vi "svx_Colormap Frequency Lines.vi"(4 "pen":T2={"Width"=1, "Style"=enum."Solid"}, 5 "Frequency Type":dbl, 6 "color(black)":u32(colorbox), 7 "plot type":T4(ring), 8 "speed profile":cluster{"time [s]":dbl[], "speed [rpm]":dbl[]} {"speed [rpm]" format="%.2f"; "time [s]" format="%.2f"}, 9 "Range":T1, 10 "Plot Area:Size":T3, 11 "picture in":picture) -> (2 "Begin":cluster{"x":i16, "y":i16}, 3 "picture Out":picture)   [LabVIEW 2017, in "SVX Colormap.xctl"]
uses:
  <vilib>/addons/_XControls/Colormap/SVX Colormap.xctl
  <vilib>/Utility/miscctls.llb/LVBoundsTypeDef.ctl
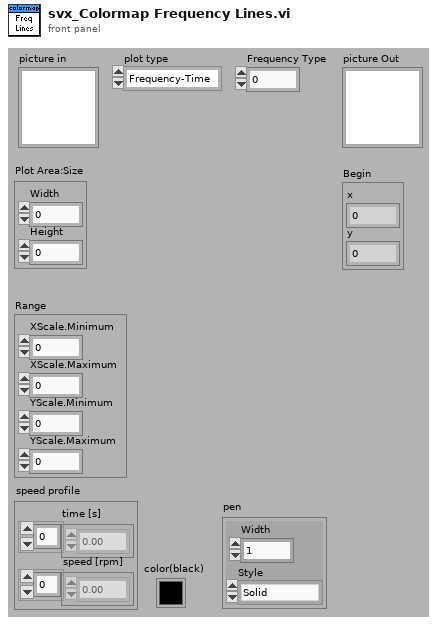
[diagram p1: front panel]
types:
  T1 = cluster{"XScale.Minimum":dbl, "XScale.Maximum":dbl, "YScale.Minimum":dbl, "YScale.Maximum":dbl}
  T2 = cluster{"Width":u16, "Style":enum32{"Solid", "Dash", "Dot", "DashDot", "DashDotDot"}}
  T3 = typedef "LVBoundsTypeDef.ctl" = cluster{"Width":u32, "Height":u32}
  T4 = enum16{"Frequency-Time", "Time-Frequency", "Order-Time", "Time-Order", "Frequency-RPM", "RPM-Frequency", "Order-RPM", "RPM-Order"}
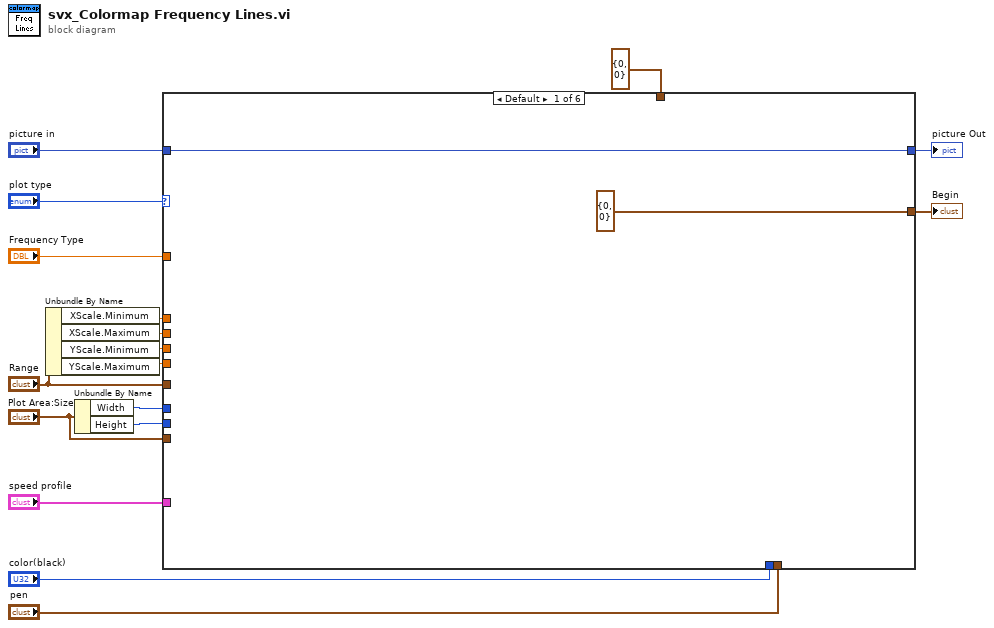
[diagram p0: block diagram]
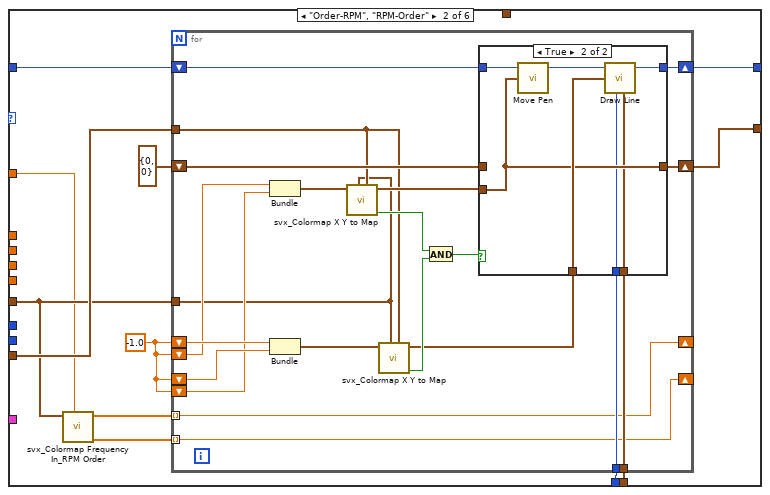
[diagram p2: hidden frame]
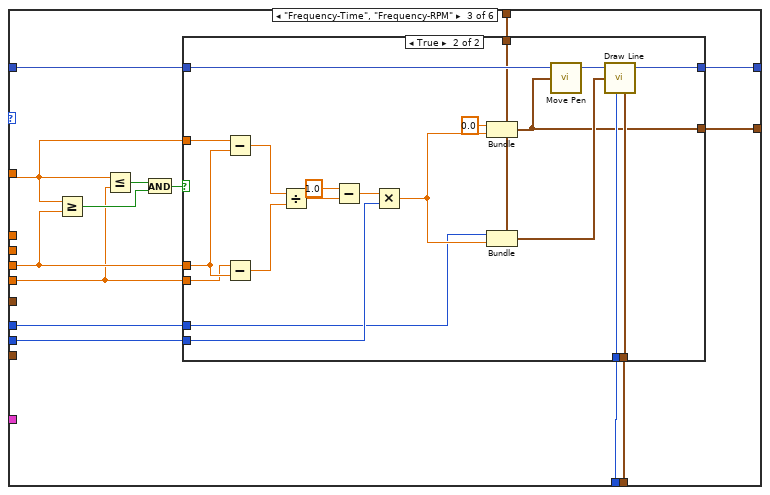
[diagram p4: hidden frame]
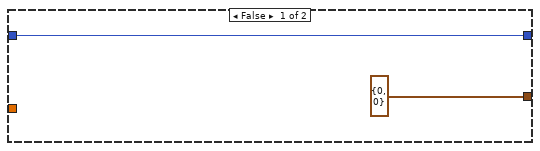
[diagram p5: hidden frame]
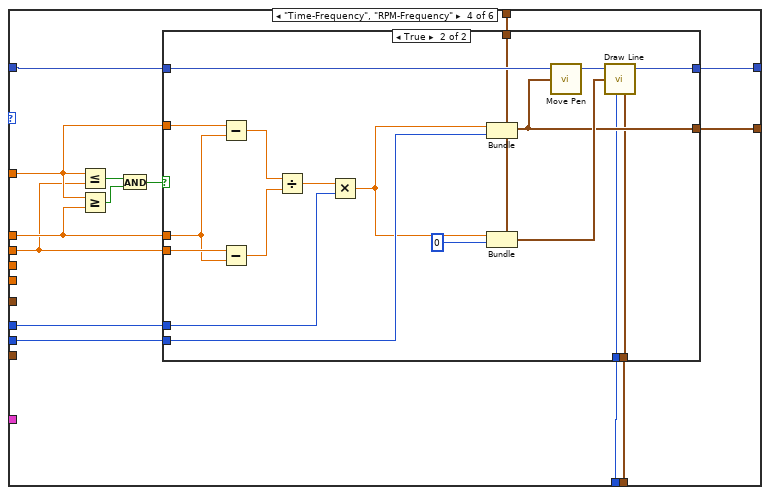
[diagram p6: hidden frame]
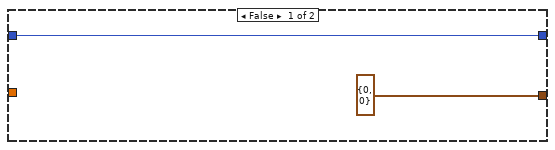
[diagram p7: hidden frame]
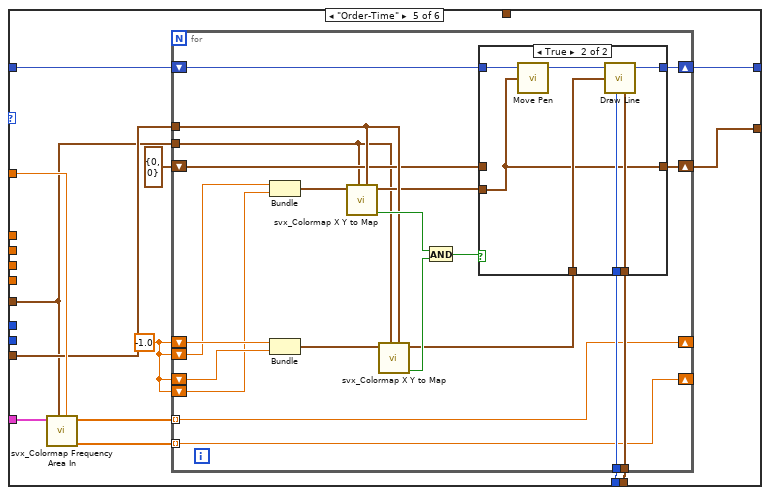
[diagram p8: hidden frame]
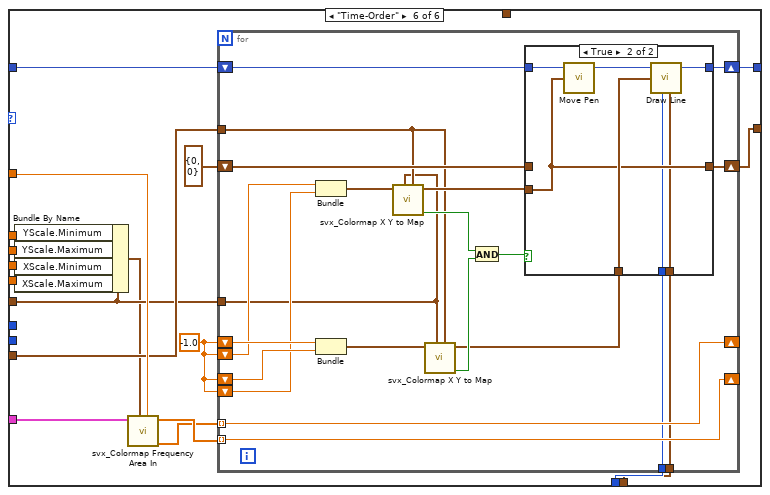
[diagram p10: hidden frame]
diagram:
  n1 = Unbundle By Name("Range") -> ("XScale.Minimum"=w15:dbl, "XScale.Maximum"=w14:dbl, "YScale.Minimum"=w13:dbl, "YScale.Maximum"=w12:dbl)
  n2 = Unbundle By Name("Plot Area:Size") -> ("Width"=w11:u32, "Height"=w10:u32)
  n3 = case shown="Default" "plot type" {
    tunnel: "Frequency Type" -> [_ w23 w72 w108 w143 w183]
    tunnel: w15 -> [_ _ _ w107 _ w187]
    tunnel: w14 -> [_ _ _ w106 _ w186]
    tunnel: w13 -> [_ _ w71 _ _ w185]
    tunnel: w12 -> [_ _ w70 _ _ w184]
    tunnel: w11 -> [_ _ w69 w105 _ _]
    tunnel: w10 -> [_ _ w68 w104 _ _]
    tunnel: [cluster{"x":i16, "y":i16} {"x"=0, "y"=0} ("Begin") w25 w63 w101 w135 w191] -> w8
    tunnel: "picture in" -> [w18 w27 w67 w102 w137 w182]
    tunnel: "color(black)" -> [_ w31 w65 w100 w142 w178]
    tunnel: "pen" -> [_ w30 w64 w99 w141 w177]
    tunnel: "speed profile" -> [_ _ _ _ w144 w190]
    tunnel: [w18 w26 w66 w103 w136 w192] -> w5
    tunnel: "Range" -> [_ w24 _ _ w132 w179]
    tunnel: "Plot Area:Size" -> [_ w29 _ _ w138 w180]
    tunnel: cluster{"x":i16, "y":i16} {"x"=0, "y"=0} ("cluster") -> [_ _ w62 w98 _ _]
    frame Default {
    }
    frame "Order-RPM", "RPM-Order" {
      w20 = -1.0 ("Numeric")
      n4 = call <vilib>:"svx_Colormap Frequency In_RPM Order.vi"("Frequency Type"=w23, "Range"=w24) -> ("Y"=w21:dbl[], "X"=w22:dbl[])  [unwired: 8 in]
      n5 = for {
        shift-right: [w49] -> w26
        shift-left: w27 -> [w48]
        shift-right: [w36] -> _
        shift-left: w20 -> [w47]
        shift-left: w20 -> [w46]
        shift-right: [w35] -> _
        shift-left: w20 -> [w45]
        shift-left: w20 -> [w44]
        shift-right: [w40] -> w25
        shift-left: cluster{"x":i16, "y":i16} {"x"=0, "y"=0} ("Map") -> [w41]
        tunnel: w29 -> [w39]
        tunnel: w24 -> [w32]
        tunnel: w31 -> [w38]
        tunnel: w30 -> [w37]
        tunnel: w22 -> [w36] mode=indexing
        tunnel: w21 -> [w35] mode=indexing
        n6 = Bundle("Numeric"=w46, "Numeric"=w44) -> (w34:cluster{"Numeric":dbl, "Numeric":dbl})  [unwired: 1 in]
        n7 = Bundle("Numeric"=w47, "Numeric"=w45) -> (w33:cluster{"Numeric":dbl, "Numeric":dbl})  [unwired: 1 in]
        n8 = call <vilib>:"svx_Colormap X Y to Map.vi"("Plot area"=w39, "Range"=w32, "cordinate"=w34) -> ("In?"=w51:bool, "Map"=w43:cluster{"x":i16, "y":i16})  [unwired: 7 in]
        n9 = call <vilib>:"svx_Colormap X Y to Map.vi"("Plot area"=w39, "Range"=w32, "cordinate"=w33) -> ("In?"=w52:bool, "Map"=w42:cluster{"x":i16, "y":i16})  [unwired: 7 in]
        n10 = And(x=w51, y=w52) -> (x .and. y?=w50:bool)
        n11 = case shown="True" w50 {
          tunnel: [w54 w59] -> w49
          tunnel: w48 -> [w54 w60]
          tunnel: w43 -> [_ w57]
          tunnel: w42 -> [_ w58]
          tunnel: w41 -> [w53 _]
          tunnel: [w53 w57] -> w40
          tunnel: w38 -> [_ w56]
          tunnel: w37 -> [_ w55]
          frame False {
          }
          frame True {
            n12 = call <vilib>:"Move Pen.vi"("new position"=w57, "picture"=w60) -> ("new picture"=w61:picture)  [unwired: 3 in]
            n13 = call <vilib>:"Draw Line.vi"("picture"=w61, "end point"=w58, "color(black)"=w56, "pen"=w55) -> ("new picture"=w59:picture)  [unwired: 5 in]
          }
        }
      }
    }
    frame "Frequency-Time", "Frequency-RPM" {
      n14 = Greater Or Equal?(x=w72, y=w71) -> (x >= y?=w74:bool)
      n15 = Less Or Equal?(x=w72, y=w70) -> (x <= y?=w75:bool)
      n16 = And(x=w75, y=w74) -> (x .and. y?=w73:bool)
      n17 = case shown="True" w73 {
        tunnel: [cluster{"x":i16, "y":i16} {"x"=0, "y"=0} ("Begin") w79] -> w63
        tunnel: w72 -> [_ w96]
        tunnel: w71 -> [_ w87]
        tunnel: w70 -> [_ w86]
        tunnel: w69 -> [_ w88]
        tunnel: w68 -> [_ w90]
        tunnel: w67 -> [w76 w84]
        tunnel: [w76 w83] -> w66
        tunnel: w65 -> [_ w81]
        tunnel: w64 -> [_ w80]
        tunnel: w62 -> [_ w78]
        frame False {
        }
        frame True {
          n18 = Subtract(x=w96, y=w87) -> (x-y=w95:dbl)
          n19 = Subtract(x=w86, y=w87) -> (x-y=w94:dbl)
          n20 = Divide(x=w95, y=w94) -> (x/y=w93:dbl)
          n21 = Subtract(x=1.0, y=w93) -> (x-y=w91:dbl)
          n22 = Multiply(x=w91, y=w90) -> (x*y=w89:dbl)
          n23 = Bundle(cluster=w78, "x"=0.0 ("Frequency Type"), "y"=w89) -> (w79:cluster{"x":i16, "y":i16})
          n24 = Bundle(cluster=w78, "x"=w88, "y"=w89) -> (w82:cluster{"x":i16, "y":i16})
          n25 = call <vilib>:"Move Pen.vi"("new position"=w79, "picture"=w84) -> ("new picture"=w85:picture)  [unwired: 3 in]
          n26 = call <vilib>:"Draw Line.vi"("picture"=w85, "end point"=w82, "color(black)"=w81, "pen"=w80) -> ("new picture"=w83:picture)  [unwired: 5 in]
        }
      }
    }
    frame "Time-Frequency", "RPM-Frequency" {
      n27 = Less Or Equal?(x=w108, y=w106) -> (x <= y?=w111:bool)
      n28 = Greater Or Equal?(x=w108, y=w107) -> (x >= y?=w110:bool)
      n29 = And(x=w111, y=w110) -> (x .and. y?=w109:bool)
      n30 = case shown="True" w109 {
        tunnel: [cluster{"x":i16, "y":i16} {"x"=0, "y"=0} ("Begin") w117] -> w101
        tunnel: w108 -> [_ w130]
        tunnel: w107 -> [_ w127]
        tunnel: w106 -> [_ w128]
        tunnel: w105 -> [_ w125]
        tunnel: w104 -> [_ w124]
        tunnel: [w112 w120] -> w103
        tunnel: w102 -> [w112 w119]
        tunnel: w100 -> [_ w116]
        tunnel: w99 -> [_ w115]
        tunnel: w98 -> [_ w114]
        frame False {
        }
        frame True {
          n31 = Subtract(x=w130, y=w127) -> (x-y=w131:dbl)
          n32 = Subtract(x=w128, y=w127) -> (x-y=w129:dbl)
          n33 = Divide(x=w131, y=w129) -> (x/y=w126:dbl)
          n34 = Multiply(x=w126, y=w125) -> (x*y=w123:dbl)
          n35 = Bundle(cluster=w114, "x"=w123, "y"=w124) -> (w117:cluster{"x":i16, "y":i16})
          n36 = Bundle(cluster=w114, "x"=w123, "y"=u32 0 ("Height")) -> (w118:cluster{"x":i16, "y":i16})
          n37 = call <vilib>:"Move Pen.vi"("new position"=w117, "picture"=w119) -> ("new picture"=w121:picture)  [unwired: 3 in]
          n38 = call <vilib>:"Draw Line.vi"("picture"=w121, "end point"=w118, "color(black)"=w116, "pen"=w115) -> ("new picture"=w120:picture)  [unwired: 5 in]
        }
      }
    }
    frame "Order-Time" {
      w133 = -1.0 ("Numeric")
      n39 = call <vilib>:"svx_Colormap Frequency Area In.vi"("Order"=w143, "Range"=w132, "speed profile"=w144) -> ("Order"=w139:dbl[], "Time(s)"=w140:dbl[])  [unwired: 7 in]
      n40 = for {
        shift-right: [w162] -> w136
        shift-left: w137 -> [w161]
        tunnel: w139 -> [w148] mode=indexing
        tunnel: w140 -> [w149] mode=indexing
        tunnel: w142 -> [w160]
        tunnel: w141 -> [w159]
        tunnel: w138 -> [w158]
        shift-right: [w149] -> _
        shift-left: w133 -> [w157]
        shift-left: w133 -> [w156]
        shift-right: [w148] -> _
        shift-left: w133 -> [w155]
        shift-left: w133 -> [w154]
        shift-right: [w146] -> w135
        shift-left: cluster{"x":i16, "y":i16} {"x"=0, "y"=0} ("Map") -> [w147]
        tunnel: w132 -> [w145]
        n41 = Bundle("Numeric"=w156, "Numeric"=w154) -> (w153:cluster{"Numeric":dbl, "Numeric":dbl})  [unwired: 1 in]
        n42 = Bundle("Numeric"=w157, "Numeric"=w155) -> (w152:cluster{"Numeric":dbl, "Numeric":dbl})  [unwired: 1 in]
        n43 = call <vilib>:"svx_Colormap X Y to Map.vi"("Plot area"=w158, "Range"=w145, "cordinate"=w153) -> ("In?"=w164:bool, "Map"=w151:cluster{"x":i16, "y":i16})  [unwired: 7 in]
        n44 = call <vilib>:"svx_Colormap X Y to Map.vi"("Plot area"=w158, "Range"=w145, "cordinate"=w152) -> ("In?"=w165:bool, "Map"=w150:cluster{"x":i16, "y":i16})  [unwired: 7 in]
        n45 = And(x=w164, y=w165) -> (x .and. y?=w163:bool)
        n46 = case shown="True" w163 {
          tunnel: [w167 w172] -> w162
          tunnel: w161 -> [w167 w173]
          tunnel: w151 -> [_ w168]
          tunnel: w160 -> [_ w171]
          tunnel: w159 -> [_ w170]
          tunnel: w150 -> [_ w169]
          tunnel: w147 -> [w166 _]
          tunnel: [w166 w168] -> w146
          frame False {
          }
          frame True {
            n47 = call <vilib>:"Move Pen.vi"("new position"=w168, "picture"=w173) -> ("new picture"=w174:picture)  [unwired: 3 in]
            n48 = call <vilib>:"Draw Line.vi"("picture"=w174, "end point"=w169, "color(black)"=w171, "pen"=w170) -> ("new picture"=w172:picture)  [unwired: 5 in]
          }
        }
      }
    }
    frame "Time-Order" {
      w188 = -1.0 ("Numeric")
      n49 = Bundle By Name(cluster=w179, "YScale.Minimum"=w187, "YScale.Maximum"=w186, "XScale.Minimum"=w185, "XScale.Maximum"=w184) -> (w175:T1)
      n50 = call <vilib>:"svx_Colormap Frequency Area In.vi"("Order"=w183, "Range"=w175, "speed profile"=w190) -> ("Order"=w176:dbl[], "Time(s)"=w189:dbl[])  [unwired: 7 in]
      n51 = for {
        shift-right: [w210] -> w192
        shift-left: w182 -> [w209]
        shift-right: [w200] -> _
        shift-left: w188 -> [w208]
        shift-left: w188 -> [w207]
        shift-right: [w199] -> _
        shift-left: w188 -> [w206]
        shift-left: w188 -> [w205]
        shift-right: [w201] -> w191
        shift-left: cluster{"x":i16, "y":i16} {"x"=0, "y"=0} ("Map") -> [w202]
        tunnel: w189 -> [w199] mode=indexing
        tunnel: w176 -> [w200] mode=indexing
        tunnel: w180 -> [w198]
        tunnel: w179 -> [w193]
        tunnel: w178 -> [w195]
        tunnel: w177 -> [w194]
        n52 = Bundle("Numeric"=w207, "Numeric"=w205) -> (w197:cluster{"Numeric":dbl, "Numeric":dbl})  [unwired: 1 in]
        n53 = Bundle("Numeric"=w208, "Numeric"=w206) -> (w196:cluster{"Numeric":dbl, "Numeric":dbl})  [unwired: 1 in]
        n54 = call <vilib>:"svx_Colormap X Y to Map.vi"("Plot area"=w198, "Range"=w193, "cordinate"=w197) -> ("In?"=w212:bool, "Map"=w204:cluster{"x":i16, "y":i16})  [unwired: 7 in]
        n55 = call <vilib>:"svx_Colormap X Y to Map.vi"("Plot area"=w198, "Range"=w193, "cordinate"=w196) -> ("In?"=w213:bool, "Map"=w203:cluster{"x":i16, "y":i16})  [unwired: 7 in]
        n56 = And(x=w212, y=w213) -> (x .and. y?=w211:bool)
        n57 = case shown="True" w211 {
          tunnel: [w215 w220] -> w210
          tunnel: w209 -> [w215 w221]
          tunnel: w204 -> [_ w218]
          tunnel: w203 -> [_ w219]
          tunnel: w202 -> [w214 _]
          tunnel: [w214 w218] -> w201
          tunnel: w195 -> [_ w217]
          tunnel: w194 -> [_ w216]
          frame False {
          }
          frame True {
            n58 = call <vilib>:"Move Pen.vi"("new position"=w218, "picture"=w221) -> ("new picture"=w222:picture)  [unwired: 3 in]
            n59 = call <vilib>:"Draw Line.vi"("picture"=w222, "end point"=w219, "color(black)"=w217, "pen"=w216) -> ("new picture"=w220:picture)  [unwired: 5 in]
          }
        }
      }
    }
  }
  "Begin" <- w8
  "picture Out" <- w5
